vi "DataReader.vi"(11 "PV html":string) -> (3 "Cluster":T1)   [LabVIEW 2020]
uses:
  <vilib>/regexp/Match Regular Expression.xnode
panel:
  out "whole match 2":string
  out "whole match":string
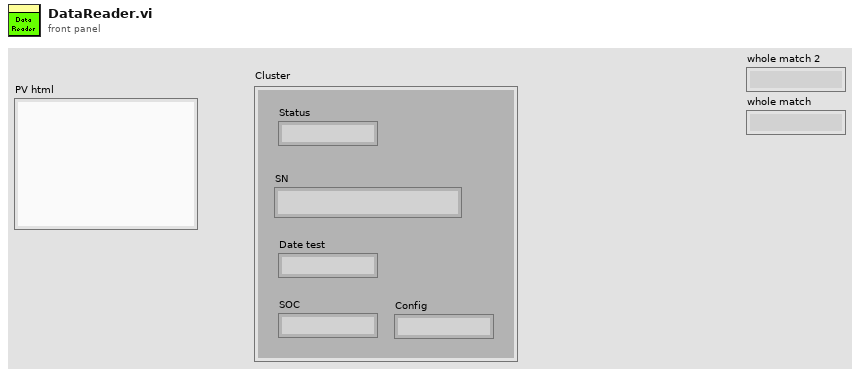
[diagram p1: front panel]
types:
  T1 = cluster{"Status":string, "SN":string, "Date test":string, "SOC":string, "Config":string}
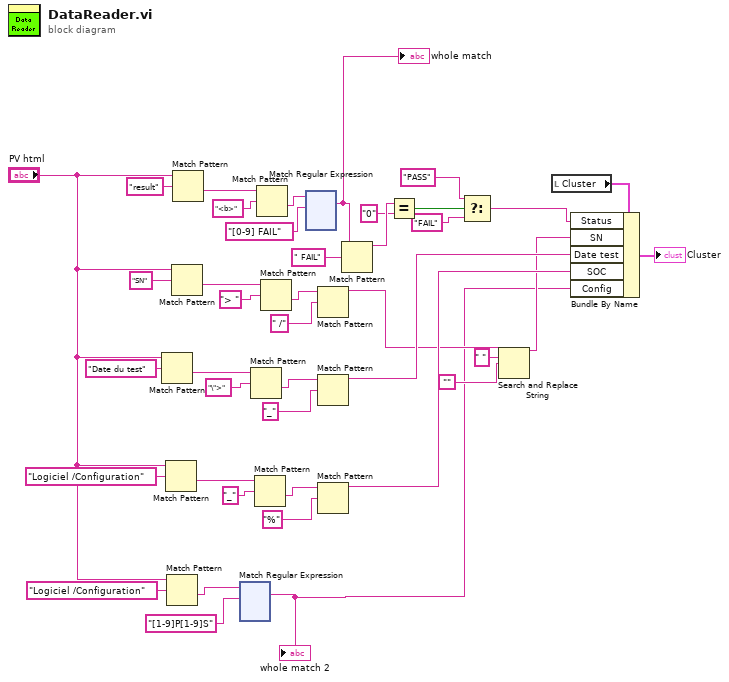
[diagram p0: block diagram]
diagram:
  n1 = Match Pattern(string="PV html", regular expression="Date du test") -> (after substring=w31:string)  [unwired: 1 in, 3 out]
  n2 = Match Pattern(string="PV html", regular expression="Logiciel /Configuration") -> (after substring=w25:string)  [unwired: 1 in, 3 out]
  n3 = Match Pattern(string="PV html", regular expression="Logiciel /Configuration") -> (after substring=w2:string)  [unwired: 1 in, 3 out]
  n4 = Match Pattern(string="PV html", regular expression="SN") -> (after substring=w37:string)  [unwired: 1 in, 3 out]
  n5 = Match Pattern(string="PV html", regular expression="result") -> (after substring=w40:string)  [unwired: 1 in, 3 out]
  n6 = xnode "Match Regular Expression"("input string"=w2, "regular expression"="[1-9]P[1-9]S") -> ("whole match"=w1:string)  [unwired: 4 in, 4 out]
  "whole match 2" <- w1
  n7 = Match Pattern(string=w31, regular expression="\">") -> (after substring=w29:string)  [unwired: 1 in, 3 out]
  n8 = Match Pattern(string=w25, regular expression="_") -> (after substring=w23:string)  [unwired: 1 in, 3 out]
  n9 = Match Pattern(string=w40, regular expression="<b>") -> (after substring=w15:string)  [unwired: 1 in, 3 out]
  n10 = Match Pattern(string=w37, regular expression="> ") -> (after substring=w35:string)  [unwired: 1 in, 3 out]
  n11 = xnode "Match Regular Expression"("input string"=w15, "regular expression"="[0-9] FAIL") -> ("whole match"=w14:string)  [unwired: 4 in, 4 out]
  "whole match" <- w14
  n12 = Match Pattern(string=w35, regular expression=" /") -> (before substring=w4:string)  [unwired: 1 in, 3 out]
  n13 = Match Pattern(string=w29, regular expression="_") -> (before substring=w26:string)  [unwired: 1 in, 3 out]
  n14 = Match Pattern(string=w23, regular expression="%") -> (before substring=w20:string)  [unwired: 1 in, 3 out]
  n15 = Match Pattern(string=w14, regular expression=" FAIL") -> (before substring=w12:string)  [unwired: 1 in, 3 out]
  n16 = Equal?(x=w12, y="0") -> (x = y?=w10:bool)
  n17 = Select(t="PASS" ("regular expression"), s=w10, f="FAIL") -> (s? t:f=w7:string)
  n18 = Search and Replace String(input string=w4, search string=" ", replace string="") -> (result string=w3:string)  [unwired: 5 in, 3 out]
  n19 = local read "Cluster"() -> (w33:T1)
  n20 = Bundle By Name(cluster=w33, "Status"=w7, "SN"=w3, "Date test"=w26, "SOC"=w20, "Config"=w1) -> (→"Cluster":T1)
